vi "Write IL Action.vi"(6 "Message Priority (Normal)":T1=enum."Normal", 8 "error in (no error)":errorcluster, 9 "Destination Enqueuer":refnum<class "Message Enqueuer.lvclass">, 10 "Actor Framework:Message":refnum<class "Message.lvclass">, 11 "IL Action in":refnum<class "IL Action.lvclass">) -> (0 "error out":errorcluster, 3 "IL Action out":refnum<class "IL Action.lvclass">)   [LabVIEW 2015, in "Interlocks.lvlib" / "IL Action.lvclass"]
uses:
  IL Action.lvclass
  <vilib>/ActorFramework/Message/Message.lvclass
  <vilib>/ActorFramework/Message Enqueuer/Message Enqueuer.lvclass
  <vilib>/ActorFramework/Message Enqueuer/Message Priority.ctl
  IL Action.lvclass/IL Action.ctl
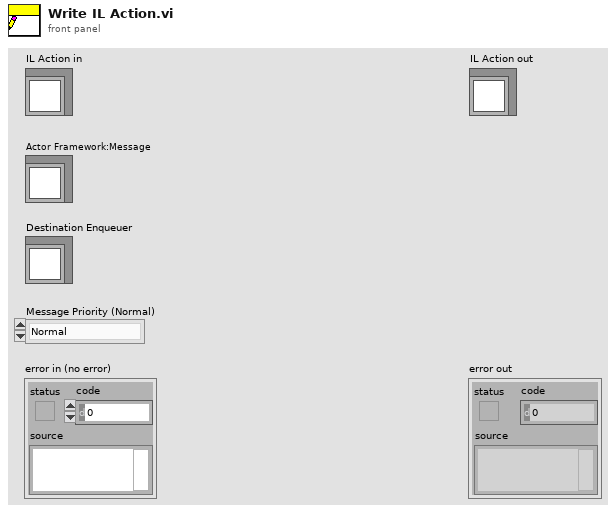
[diagram p1: front panel]
types:
  T1 = typedef "Actor Framework.lvlib/Message Enqueuer.lvclass/Message Priority.ctl" = enum16{"Low", "Normal", "High"}
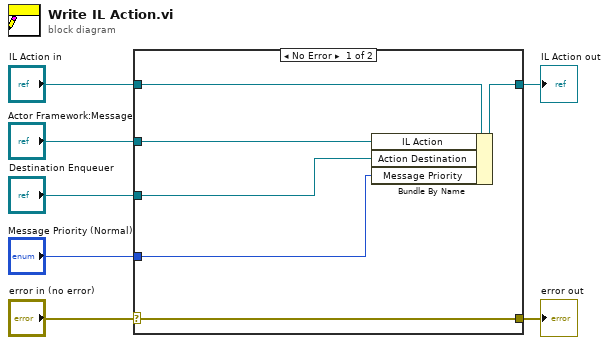
[diagram p0: block diagram]
diagram:
  n1 = case shown="No Error" "error in (no error)" {
    selector: "error in (no error)" -> [w13 w14]
    tunnel: [w13 w14] -> w6
    tunnel: [w11 w15] -> w4
    tunnel: "IL Action in" -> [w12 w15]
    tunnel: "Actor Framework:Message" -> [w10 _]
    tunnel: "Destination Enqueuer" -> [w9 _]
    tunnel: "Message Priority (Normal)" -> [w8 _]
    frame No Error {
      n2 = Bundle By Name(cluster=w12, "IL Action"=w10, "Action Destination"=w9, "Message Priority"=w8) -> (w11:refnum<class "IL Action.lvclass">)
    }
    frame Error {
    }
  }
  "error out" <- w6
  "IL Action out" <- w4
